vi "kick.vi"(5 "kick_z":dbl, 6 "KickTarget":dbl[](array[numeric]), 7 "kick_x":dbl, 8 "error in (no error)":errorcluster, 9 "Ball":refnum<class "Ball.lvclass">, 10 "Robot":refnum<class "Robot.lvclass">, 11 "KickToSkill in":refnum<class "KickToSkill.lvclass">) -> (0 "error out":errorcluster, 2 "Robot out":refnum<class "Robot.lvclass">, 3 "KickToSkill out":refnum<class "KickToSkill.lvclass">)   [LabVIEW 2023, in "KickToSkill.lvclass"]
uses:
  KickToSkill.lvclass
  Robot_class/Robot.lvclass
  Ball_class/Ball.lvclass
  C:/Users/ebert/Desktop/roboime/SSL_AI/Object_class/Object.lvclass
  Game_class/Navigation/driveMode.ctl
  KickToSkill.lvclass/KickToSkill.ctl
  Object_class/Object.lvclass/Object.ctl
  Robot_class/Robot.lvclass/Robot.ctl
  <vilib>/Analysis/baseanly.llb/Unit Vector (DBL).vi
  Object_class/Read position(x,y).vi
  Read WaitKick.vi
  Robot_class/Write dest_x.vi
  Robot_class/Write dest_y.vi
  Robot_class/Write dest_orientation.vi
  Robot_class/Write kick_x.vi
  Robot_class/Write kick_z.vi
  <vilib>/Analysis/NI_AALBase.lvlib
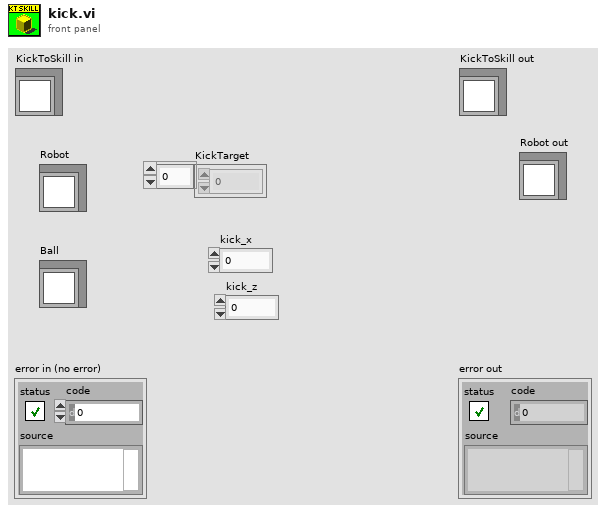
[diagram p1: front panel]
types:
  T1 = typedef "driveMode.ctl" = enum16{"Fast", "SafeDrive"}
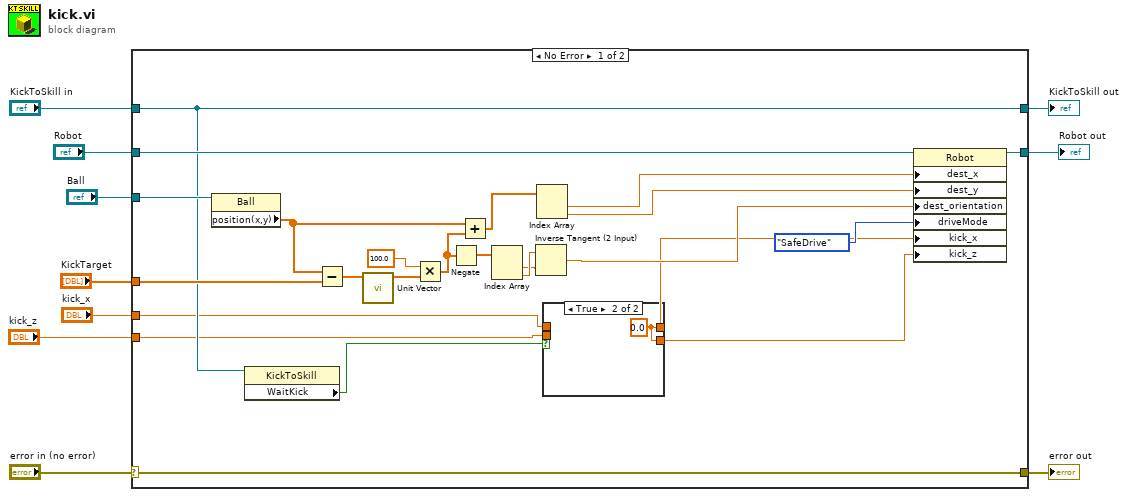
[diagram p0: block diagram]
diagram:
  n1 = case shown="No Error" "error in (no error)" {
    selector: "error in (no error)" -> [w34 w40]
    tunnel: [w34 w40] -> w9
    tunnel: [w16 w39] -> w7
    tunnel: "KickToSkill in" -> [w16 w39]
    tunnel: "Robot" -> [w18 w38]
    tunnel: [w33 w38] -> w5
    tunnel: "Ball" -> [w22 _]
    tunnel: "KickTarget" -> [w19 _]
    tunnel: "kick_x" -> [w14 _]
    tunnel: "kick_z" -> [w13 _]
    frame No Error {
      n2 = property class="Ball"(reference=w22) -> ("position(x,y)"=w30:dbl[])  [unwired: 1 in, 2 out]
      n3 = property class="KickToSkill"(reference=w16) -> ("WaitKick"=w15:bool)  [unwired: 1 in, 2 out]
      n4 = Subtract(x=w30, y=w19) -> (x-y=w31:dbl[])
      n5 = call-poly <vilib>:"Unit Vector.vi"("Input Vector"=w31) -> ("Unit Vector"=w28:dbl[])  [unwired: 8 in, 2 out]
      n6 = Multiply(x=100.0, y=w28) -> (x*y=w24:dbl[])
      n7 = Negate(x=w24) -> (-x=w23:dbl[])
      n8 = Add(x=w30, y=w24) -> (x+y=w27:dbl[])
      n9 = Index Array(array=w23) -> (element #1=w25:dbl, element #2=w26:dbl)  [unwired: 2 in]
      n10 = Inverse Tangent (2 Input)(1:w25, 2:w26) -> (0:w17:dbl)
      n11 = Index Array(array=w27) -> (element #1=w21:dbl, element #2=w20:dbl)  [unwired: 2 in]
      n12 = case shown="True" w15 {
        tunnel: w14 -> [w36 _]
        tunnel: w13 -> [w35 _]
        tunnel: [w36 w37] -> w12
        tunnel: [w35 w37] -> w11
        frame False {
        }
        frame True {
          w37 = 0.0 ("kick_x")
        }
      }
      n13 = property class="Robot"(reference=w18, "dest_x"=w21, "dest_y"=w20, "dest_orientation"=w17, "driveMode"=driveMode."SafeDrive", "kick_x"=w12, "kick_z"=w11) -> (reference out=w33:refnum<class "Robot.lvclass">)  [unwired: 1 in, 1 out]
    }
    frame Error {
    }
  }
  "error out" <- w9
  "KickToSkill out" <- w7
  "Robot out" <- w5
